vi "Env AE.vi"(1 "Set Value":refnum<k24>) -> (0 "Env":refnum<k24>)   [LabVIEW 2025]
uses:
  C:/Users/Simon/Documents/GitHub/LV-WebView2/Source/Libs/Microsoft.Web.WebView2.Core.dll
  Libs/Microsoft.Web.WebView2.Core.dll
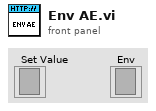
[diagram p1: front panel]
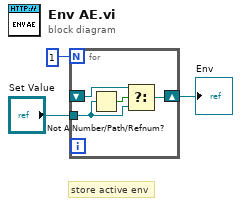
[diagram p0: block diagram]
diagram:
  # "store active env"
  n1 = for {
    N: 1 -> [_]
    tunnel: "Set Value" -> [w6]
    shift-right: [w5] -> w1
    shift-left: _ -> [w4]
    n2 = Not A Number/Path/Refnum?(number/path/refnum=w6) -> (NaN/Path/Refnum?=w7:bool)
    n3 = Select(t=w4, s=w7, f=w6) -> (s? t:f=w5:refnum<k24>)
  }
  "Env" <- w1
